vi "SVXMPL_Continuous Broadband Waveform.vi"(5 "signal type":T1(ring)=enum."Uniform white noise", 6 "sampling info":cluster{"Fs":dbl, "#s":dbl}={"Fs"=1000.0, "#s"=1000.0} {"#s" format="%.2p"; "Fs" format="%.2p"}, 7 "generation control":T2(ring), 8 "error in":errorcluster, 9 "delay until transition (0 samples)":i32, 10 "initial waveform state":cluster{"amplitude":dbl, "offset":dbl, "tf":dbl} {"tf" format="%.2f"; "offset" format="%.2f"; "amplitude" format="%.2f"}, 11 "desired waveform state":T3={"amplitude"=1.0, "offset"=0.0, "tf (ignored)"=0.0} {"tf (ignored)" format="%.2f"; "offset" format="%.2p"; "amplitude" format="%.2p"}) -> (0 "error out":errorcluster, 1 "index of transition":i32, 2 "final waveform state":cluster{"amplitude":dbl, "offset":dbl, "tf":dbl} {"tf" format="%.2f"; "offset" format="%.2f"; "amplitude" format="%.2f"}, 3 "signal out":waveform(dbl))   [LabVIEW 2017]
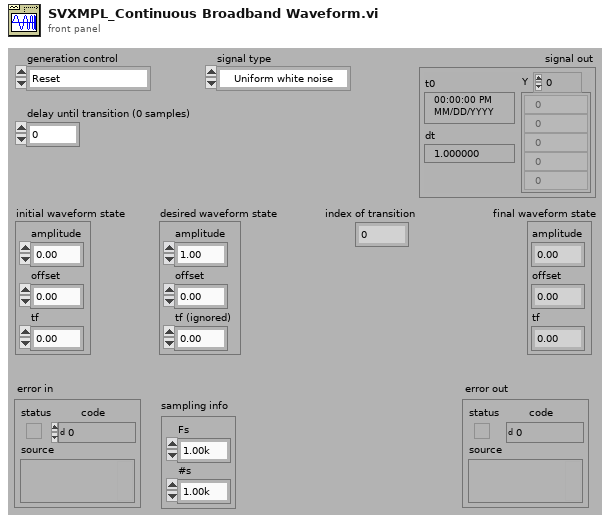
[diagram p1: front panel]
types:
  T1 = enum16{"Sine wave", "Dual tone (IMD)", "Multitone", "Chirp", "Frequency flat chirp", "Uniform white noise", "Gaussian white noise", "Pink noise", "PRN"}
  T2 = enum16{"Reset", "Continue from previous", "Continue from state", "Zero from previous", "Zero from state"}
  T3 = cluster{"amplitude":dbl, "offset":dbl, "tf (ignored)":dbl}
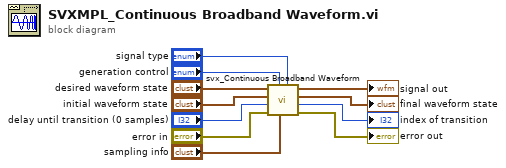
[diagram p0: block diagram]
diagram:
  n1 = call <vilib>:"svx_Continuous Broadband Waveform.vi"("signal type"="signal type", "sampling info"="sampling info", "generation control"="generation control", "error in"="error in", "delay until transition (0 samples)"="delay until transition (0 samples)", "initial waveform state"="initial waveform state", "desired waveform state"="desired waveform state") -> ("error out"=→"error out":errorcluster, "index of transition"=→"index of transition":i32, "final waveform state"=→"final waveform state":cluster{"amplitude":dbl, "offset":dbl, "tf":dbl}, "signal out"=→"signal out":waveform(dbl))  [unwired: 1 in]
